vi "Get Key Points.vi"(1 "Path":i32[][](array[numeric])) -> (0 "Key Points":i32[][](array[numeric]))   [LabVIEW 2015]
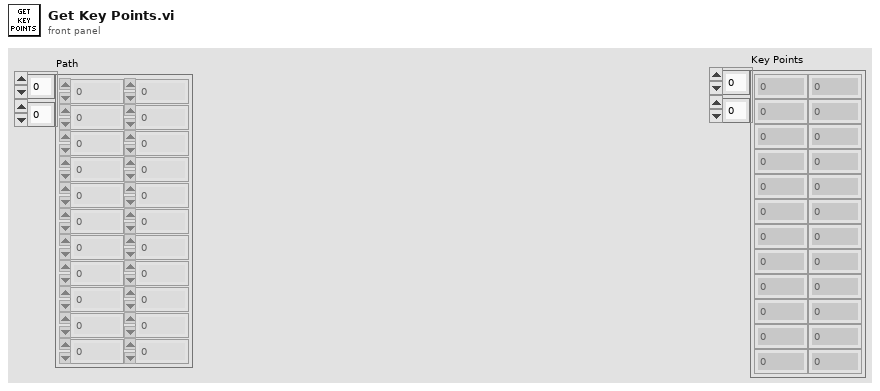
[diagram p1: front panel]
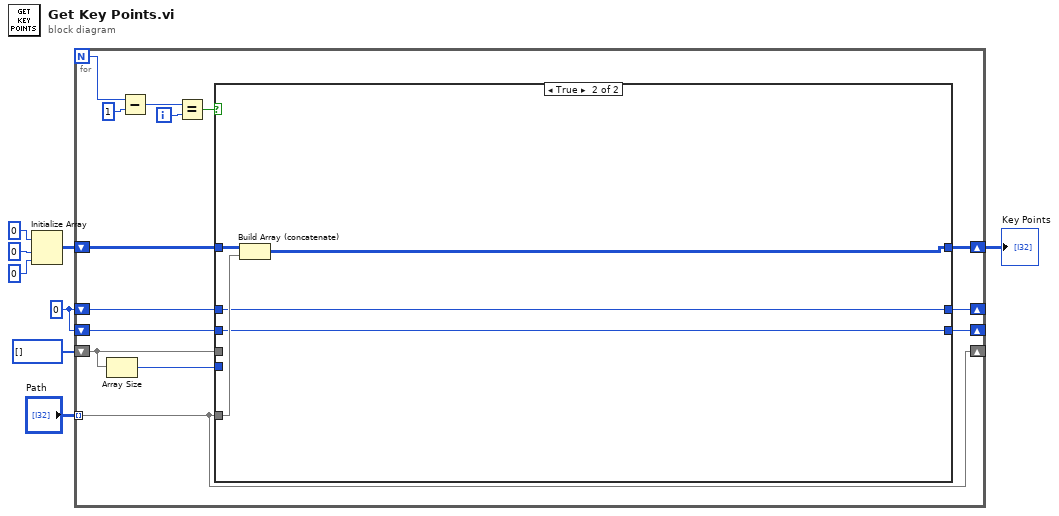
[diagram p0: block diagram]
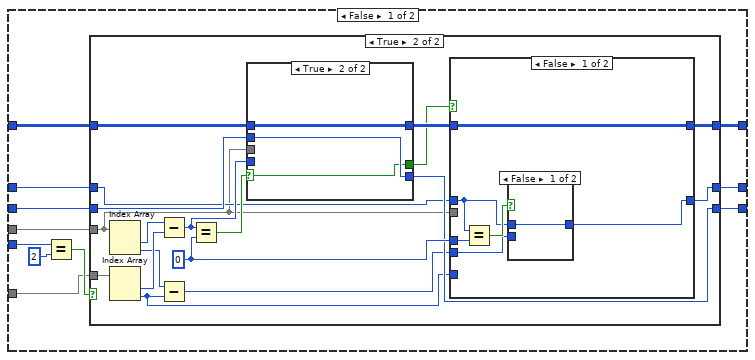
[diagram p2: hidden frame]
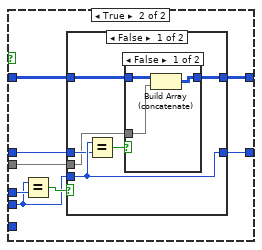
[diagram p5: hidden frame]
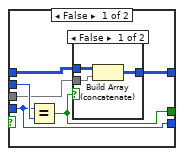
[diagram p8: hidden frame]
diagram:
  w1 = 0
  n1 = Initialize Array(0, 0 ("dimension size"), 0 ("dimension size")) -> (w4:i32[][])
  n2 = for {
    N -> [w11]
    tunnel: "Path" -> [w20] mode=indexing
    shift-right: [w20] -> _
    shift-left: i32[] [] ("Path") -> [w21]
    shift-right: [w19] -> _
    shift-left: w1 -> [w18]
    shift-right: [w16] -> w3
    shift-left: w4 -> [w17]
    shift-right: [w15] -> _
    shift-left: w1 -> [w14]
    i -> [w13]
    n3 = Array Size(array=w21) -> (size(s)=w22:i32)
    n4 = Subtract(x=w11, y=1) -> (x-y=w9:i32)
    n5 = Equal?(x=w9, y=w13) -> (x = y?=w12:bool)
    n6 = case shown="True" w12 {
      tunnel: w22 -> [w33 _]
      tunnel: w21 -> [w30 _]
      tunnel: w20 -> [w29 w99]
      tunnel: [w28 w97] -> w19
      tunnel: w18 -> [w27 w97]
      tunnel: w17 -> [w26 w100]
      tunnel: [w25 w98] -> w16
      tunnel: [w24 w96] -> w15
      tunnel: w14 -> [w23 w96]
      frame False {
        n7 = Equal?(x=w33, y=2) -> (x = y?=w31:bool)
        n8 = case shown="True" w31 {
          tunnel: w30 -> [_ w41]
          tunnel: w29 -> [_ w42]
          tunnel: [w35 w48] -> w28
          tunnel: w27 -> [w35 w49]
          tunnel: w26 -> [w34 w47]
          tunnel: [w34 w44] -> w25
          tunnel: [w36 w46] -> w24
          tunnel: w23 -> [w36 w45]
          frame False {
          }
          frame True {
            w52 = 0 ("y")
            n9 = Index Array(array=w41) -> (element #1=w54:i32, element #2=w38:i32)  [unwired: 2 in]
            n10 = Index Array(array=w42) -> (element #1=w53:i32, element #2=w39:i32)  [unwired: 2 in]
            n11 = Subtract(x=w54, y=w53) -> (x-y=w50:i32)
            n12 = Subtract(x=w38, y=w39) -> (x-y=w37:i32)
            n13 = Equal?(x=w50, y=w52) -> (x = y?=w51:bool)
            n14 = case shown="True" w51 {
              selector: w51 -> [_ w93]
              tunnel: w50 -> [w87 _]
              tunnel: w49 -> [w88 w95]
              tunnel: [w87 w95] -> w48
              tunnel: w47 -> [w86 w94]
              tunnel: [w85 w94] -> w43
              tunnel: w41 -> [w84 _]
              tunnel: [w83 w93] -> w40
              frame False {
                n15 = Equal?(x=w87, y=w88) -> (x = y?=w83:bool)
                n16 = case shown="False" w83 {
                  tunnel: w86 -> [w91 w92]
                  tunnel: [w89 w92] -> w85
                  tunnel: w84 -> [w90 _]
                  frame False {
                    n17 = Build Array (concatenate)(w91, w90) -> (w89:i32[][])
                  }
                  frame True {
                  }
                }
              }
              frame True {
              }
            }
            n18 = case shown="False" w40 {
              tunnel: w39 -> [_ _]
              tunnel: w52 -> [w59 w70]
              tunnel: [w57 w68] -> w46
              tunnel: w45 -> [w55 w67]
              tunnel: [w60 w66] -> w44
              tunnel: w43 -> [w60 w65]
              tunnel: w41 -> [_ w64]
              tunnel: w37 -> [w56 w63]
              frame False {
                n19 = Equal?(x=w55, y=w59) -> (x = y?=w58:bool)
                n20 = case shown="False" w58 {
                  tunnel: [w61 w62] -> w57
                  tunnel: w56 -> [_ w62]
                  tunnel: w55 -> [w61 _]
                  frame False {
                  }
                  frame True {
                  }
                }
              }
              frame True {
                n21 = Equal?(x=w63, y=w70) -> (x = y?=w69:bool)
                n22 = case shown="False" w69 {
                  tunnel: w63 -> [w76 _]
                  tunnel: [w76 w81] -> w68
                  tunnel: w67 -> [w75 w81]
                  tunnel: [w73 w82] -> w66
                  tunnel: w65 -> [w72 w82]
                  tunnel: w64 -> [w71 _]
                  frame False {
                    n23 = Equal?(x=w76, y=w75) -> (x = y?=w74:bool)
                    n24 = case shown="False" w74 {
                      tunnel: [w77 w80] -> w73
                      tunnel: w72 -> [w79 w80]
                      tunnel: w71 -> [w78 _]
                      frame False {
                        n25 = Build Array (concatenate)(w79, w78) -> (w77:i32[][])
                      }
                      frame True {
                      }
                    }
                  }
                  frame True {
                  }
                }
              }
            }
          }
        }
      }
      frame True {
        n26 = Build Array (concatenate)(w100, w99) -> (w98:i32[][])
      }
    }
  }
  "Key Points" <- w3
